vi "FPGA Start FIFO By Name.vi"(8 "error in (no error)":errorcluster, 10 "FIFO":string, 11 "FPGA Session In":refnum<class "FPGA Interface Base.lvclass">) -> (0 "error out":errorcluster, 3 "FPGA Session Out":refnum<class "FPGA Interface Base.lvclass">)   [LabVIEW 2010, in "FPGA Interface Base.lvclass"]
doc: "Starts a FIFO."
uses:
  <userlib>/_FPGA Interface Advanced Tools/FPGA Interface Base/FPGA Interface Base.lvclass
  <userlib>/_FPGA Interface Advanced Tools/FPGA Interface Base/FPGA Interface Base.lvclass/FPGA Interface Base.ctl
  <vilib>/Utility/error.llb/Error Cluster From Error Code.vi
  <userlib>/_FPGA Interface Advanced Tools/FPGA Interface Base/Accessors/FPGA Read Session.vi
  <userlib>/_FPGA Interface Advanced Tools/FPGA Interface Wrapper/FPGA Interface Wrapper.lvlib
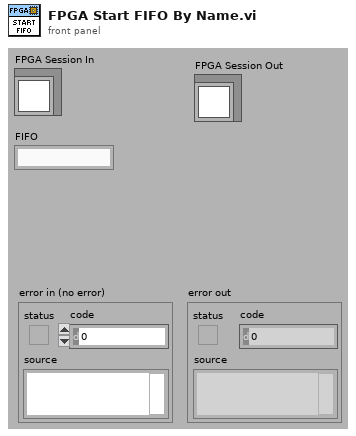
[diagram p1: front panel]
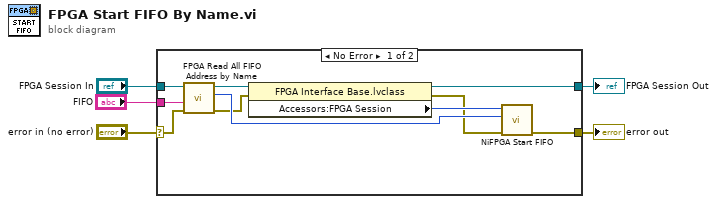
[diagram p0: block diagram]
diagram:
  n1 = case shown="No Error" "error in (no error)" {
    selector: "error in (no error)" -> [w14 w17]
    tunnel: [w6 w17] -> w1
    tunnel: [w7 w16] -> w2
    tunnel: "FPGA Session In" -> [w15 w16]
    tunnel: "FIFO" -> [w13 _]
    frame No Error {
      n2 = call <userlib>:"FPGA Read All FIFO Address by Name.vi"("error in (no error)"=w14, "Name"=w13, "FPGA Interface Base in"=w15) -> ("error out"=w10:errorcluster, "Address"=w12:u32, "FPGA Interface Base out"=w11:refnum<class "FPGA Interface Base.lvclass">)  [unwired: 5 in, 1 out]
      n3 = property class="FPGA Interface Base.lvclass"(reference=w11, error in=w10) -> (reference out=w7:refnum<class "FPGA Interface Base.lvclass">, error out=w8:errorcluster, "Accessors:FPGA Session"=w9:u32)
      n4 = call <userlib>:"NiFPGA Start FIFO.vi"("error in (no error)"=w8, "FIFO"=w12, "Session"=w9) -> ("error out"=w6:errorcluster)  [unwired: 7 in, 1 out]
    }
    frame Error {
    }
  }
  "error out" <- w1
  "FPGA Session Out" <- w2
